vi "Login Candidate.vi"(0 "Candidate ID":string, 5 "Password":string, 11 "error in (no error)":errorcluster) -> (4 "LoggedIn":bool, 15 "error out":errorcluster)   [LabVIEW 2014, in "Coding Platform.lvlib"]
uses:
  Coding Platform.lvlib
  Typedefs/User Event Operations.ctl
  Datatypes/Login.ctl
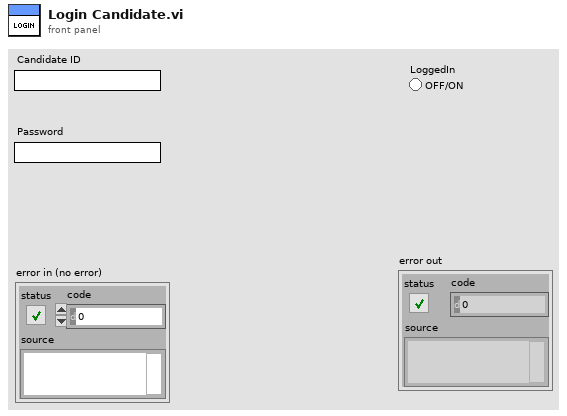
[diagram p1: front panel]
types:
  T1 = typedef "Coding Platform.lvlib/Login.ctl" = cluster{"Candidate_ID":string, "Password":string, "notifier":refnum<notifier>}
  T2 = typedef "Coding Platform.lvlib/User Event Operations.ctl" = enum16{"Create", "Genereate", "Destroy", "Get Reference"}
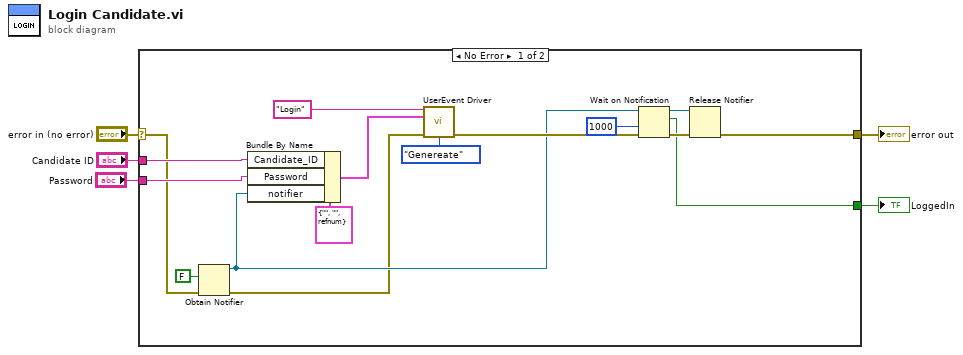
[diagram p0: block diagram]
diagram:
  n1 = case shown="No Error" "error in (no error)" {
    selector: "error in (no error)" -> [w6 w22]
    tunnel: [w10 w22] -> w5
    tunnel: "Candidate ID" -> [w16 _]
    tunnel: "Password" -> [w15 _]
    tunnel: [w8 _] -> w1
    frame No Error {
      n2 = Obtain Notifier(notification data type=FALSE, error in (no error)=w6) -> (notifier out=w13:refnum<notifier>, error out=w7:errorcluster)  [unwired: 2 in, 1 out]
      n3 = Bundle By Name(cluster=T1 {"Candidate_ID"="", "Password"="", "notifier"=refnum} ("Login"), "Candidate_ID"=w16, "Password"=w15, "notifier"=w13) -> (w17:T1)
      n4 = call "UserEvent Driver.vi"("Message"="Login", "Data"=w17, "error in (no error)"=w7, "Operations(Get Reference)"=User_Event_Operations."Genereate") -> ("error out"=w21:errorcluster)  [unwired: 10 in, 1 out]
      n5 = Wait on Notification(notifier=w13, timeout in ms (-1)=1000, error in (no error)=w21) -> (notifier out=w9:refnum<notifier>, notification=w8:bool, error out=w14:errorcluster)  [unwired: 1 in, 1 out]
      n6 = Release Notifier(notifier=w9, error in (no error)=w14) -> (error out=w10:errorcluster)  [unwired: 1 in, 2 out]
    }
    frame Error {
    }
  }
  "error out" <- w5
  "LoggedIn" <- w1
